vi "Read.vi"(11 "Error Result in":refnum<class "Error Result.lvclass">) -> (2 "Error":errorcluster)   [LabVIEW 2020, in "Promises.lvlib" / "Error Result.lvclass"]
uses:
  Error Result.lvclass
  Error Result.lvclass/Error Result.ctl
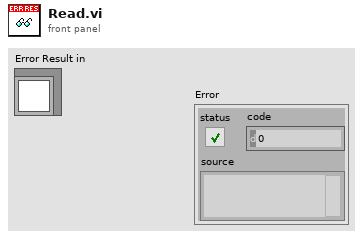
[diagram p1: front panel]
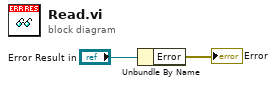
[diagram p0: block diagram]
diagram:
  n1 = Unbundle By Name("Error Result in") -> ("Error"=→"Error":errorcluster)
